vi "nowy NUMBER rozny od poprzedniego.vi"(4 "Numeric":dbl) -> (1 "x != y?":bool)   [LabVIEW 2015, in "Biblioteka moduł map v3.lvlib" / "task erl.lvlib"]
uses:
  TASK ERL/task erl.lvlib
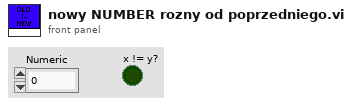
[diagram p1: front panel]
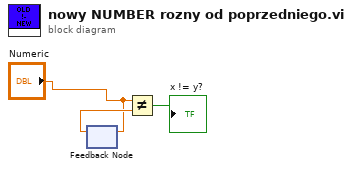
[diagram p0: block diagram]
diagram:
  n1 = feedback #1() -> (w2:dbl)  [unwired: 1 in]
  n2 = feedback-in #1("Numeric") -> ()
  n3 = Not Equal?(x="Numeric", y=w2) -> (x != y?=→"x != y?":bool)
